vi "MT Measure Quadrature Impairments.vi"   [LabVIEW 2020, in "niDMT.lvlib"]
doc: "Measures and reports quadrature impairments over a single user-specified window for each of the supported modulation types. This VI must be called once for each measurement window."
uses:
  <vilib>/addons/Modulation/niDMT.lvlib
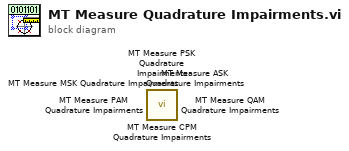
[diagram p0: block diagram]
diagram:
  n1 = call <vilib>:"MT Measure CPM Quadrature Impairments.vi"() -> ()  [unwired: 8 in, 8 out]
  n2 = call <vilib>:"MT Measure ASK Quadrature Impairments.vi"() -> ()  [unwired: 10 in, 6 out]
  n3 = call <vilib>:"MT Measure PAM Quadrature Impairments.vi"() -> ()  [unwired: 10 in, 6 out]
  n4 = call <vilib>:"MT Measure QAM Quadrature Impairments.vi"() -> ()  [unwired: 8 in, 8 out]
  n5 = call <vilib>:"MT Measure MSK Quadrature Impairments.vi"() -> ()  [unwired: 8 in, 8 out]
  n6 = call <vilib>:"MT Measure PSK Quadrature Impairments.vi"() -> ()  [unwired: 8 in, 8 out]
